vi "Initialize Date.vi"(8 "error in (no error)":errorcluster, 11 "Budgetizer in":refnum<class "Budgetizer.lvclass">) -> (0 "error out":errorcluster, 3 "Budgetizer out":refnum<class "Budgetizer.lvclass">)   [LabVIEW 2018, in "Budgetizer.lvclass"]
uses:
  Budgetizer.lvclass
  Budgetizer.lvclass/Budgetizer.ctl
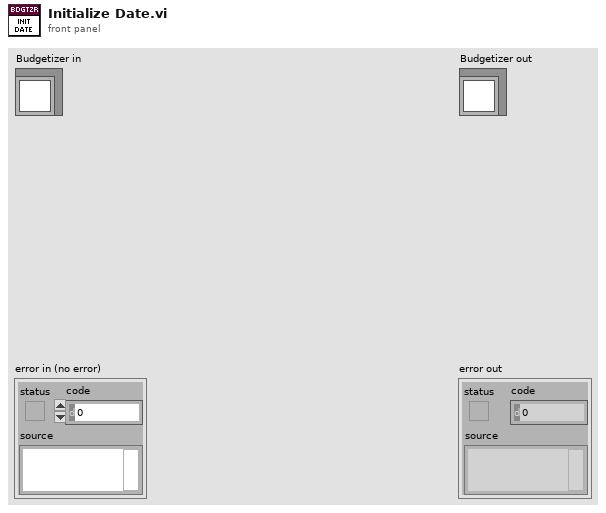
[diagram p1: front panel]
types:
  T1 = typedef "LVDateTimeRec.ctl" = cluster{"fractional second":dbl, "second":i32, "minute":i32, "hour":i32, "day of month":i32, "month":i32, "year":i32, "day of week":i32, "day of year":i32, "DST":i32}
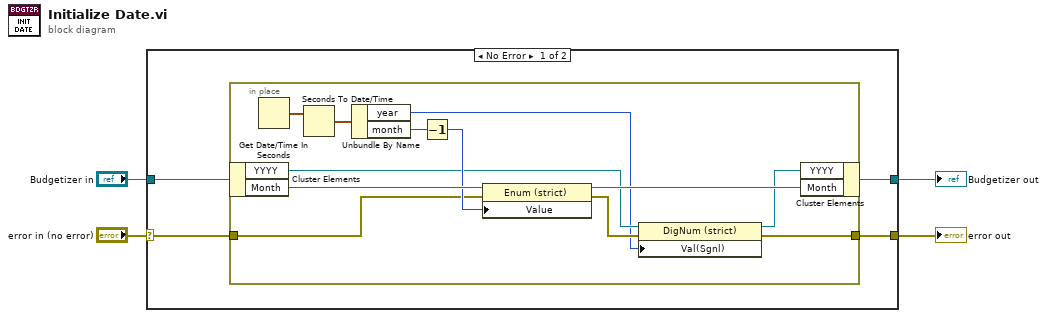
[diagram p0: block diagram]
diagram:
  n1 = case shown="No Error" "error in (no error)" {
    selector: "error in (no error)" -> [w7 w22]
    tunnel: [w6 w22] -> w3
    tunnel: [w5 w21] -> w1
    tunnel: "Budgetizer in" -> [w8 w21]
    frame No Error {
      n2 = in-place {
        in-place-border: w7 -> [w14]
        in-place-border: [w9] -> w6
        n3 = in-place-cluster #1(w8) -> ("YYYY"=w13:refnum<vi>, "Month"=w17:refnum<vi>)
        n4 = Get Date/Time In Seconds() -> (seconds since 1Jan1904=w18:timestamp)
        n5 = Seconds To Date/Time(time stamp (now)=w18) -> (date time rec=w19:T1)  [unwired: 1 in]
        n6 = Unbundle By Name(w19) -> ("year"=w10:i32, "month"=w20:i32)
        n7 = Decrement(x=w20) -> (x-1=w16:i32)
        n8 = property class="Enum (strict)"(reference=w17, error in=w14, "Value"=w16) -> (reference out=w15:refnum<vi>, error out=w12:errorcluster)
        n9 = property class="DigNum (strict)"(reference=w13, error in=w12, "Val(Sgnl)"=w10) -> (reference out=w11:refnum<vi>, error out=w9:errorcluster)
        n10 = in-place-cluster #1("YYYY"=w11, "Month"=w15) -> (w5:refnum<class "Budgetizer.lvclass">)
      }
    }
    frame Error {
    }
  }
  "error out" <- w3
  "Budgetizer out" <- w1
